vi "ConfigDlg.vi"(8 "error in (no error)":errorcluster, 11 "AnalysisPluginsBase in":refnum<class "AnalysisPluginsBase.lvclass">) -> (0 "error out":errorcluster, 2 "Changed":bool, 3 "AnalysisPluginsBase out":refnum<class "AnalysisPluginsBase.lvclass">)   [LabVIEW 2014, in "AnalysisPlugins.lvlib" / "AnalysisPluginsBase.lvclass"]
uses:
  AnalysisPluginsBase.lvclass
  Typedefs/clAnalysisConfig.ctl
  AnalysisPluginsBase.lvclass/AnalysisPluginsBase.ctl
  <userlib>/NIST/BaseClasses/BasePlugin_class/BasePlugin.lvclass/BasePlugin.ctl
  <userlib>/NIST/BaseClasses/BasePlugin_class/Accessors/Read PluginIniFilePath.vi
  Accessors/Write clConfig.vi
  Accessors/Read clConfig.vi
  Accessors/Read DelayCorr.vi
  Accessors/Read MagCorr.vi
  <vilib>/Utility/config.llb/NI_LVConfig.lvlib
panel:
  in  "BtnCancel":bool
  in  "MagCorr":dbl[](array[numeric])
  in  "DelayCorr":dbl[](array[numeric])
  in  "clAnalysisConfig":T1={"F0"=60, "SettlingTime"=7.0, "AnalysisCycles"=20.0, "SampleRate"=4800.0, "NumChannels"=6, "TsOffset"=enum."start"}
  in  "btnDone":bool
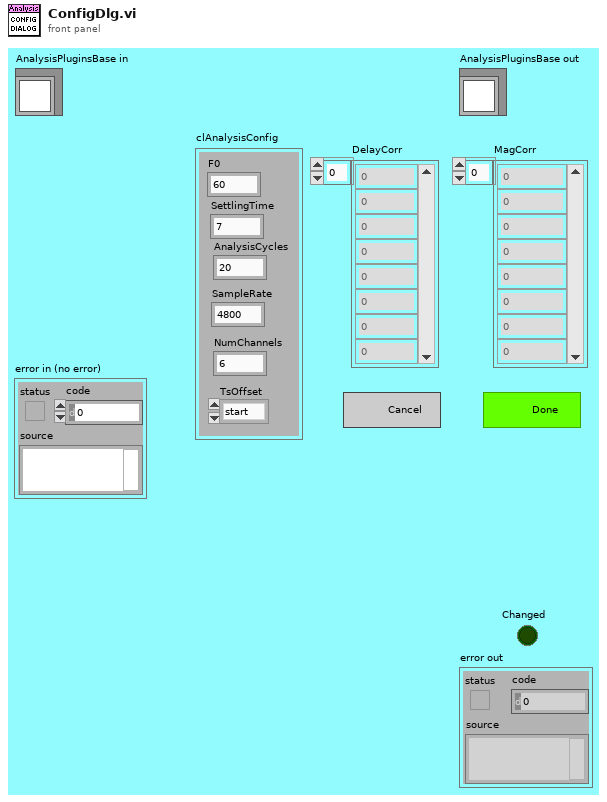
[diagram p1: front panel]
types:
  T1 = typedef "AnalysisPlugins.lvlib/AnalysisPluginsBase.lvclass/clAnalysisConfig.ctl" = cluster{"F0":u32, "SettlingTime":dbl, "AnalysisCycles":dbl, "SampleRate":dbl, "NumChannels":u32, "TsOffset":enum16{"start", "middle", "end"}}
  T2 = enum32{"Invalid", "Standard", "Closed", "Hidden", "Minimized", "Maximized"}
  T3 = enum32{"Invalid", "Default", "Floating", "Floating/Auto-Hide", "Modal"}
  T4 = typedef "NI_LVConfig.lvlib/Config Data RefNum.ctl" = refnum<k1>
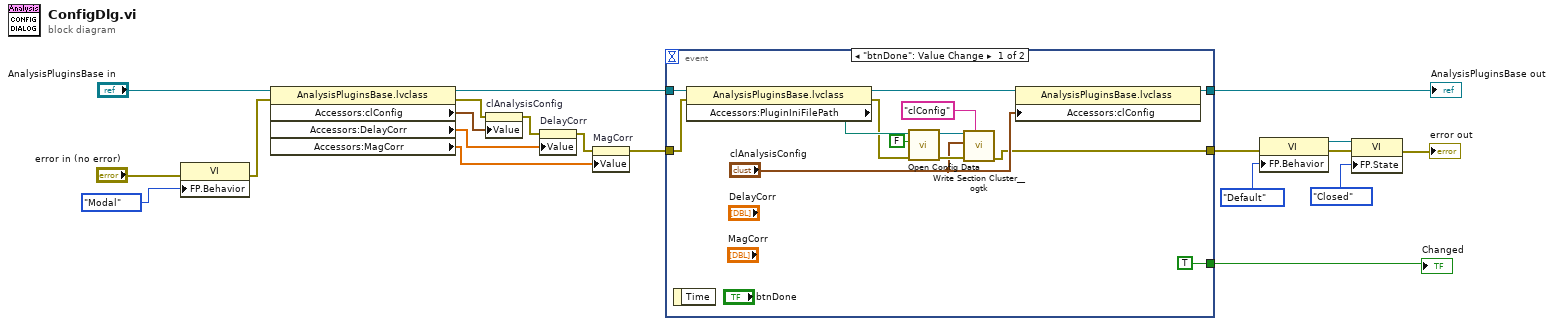
[diagram p0: block diagram]
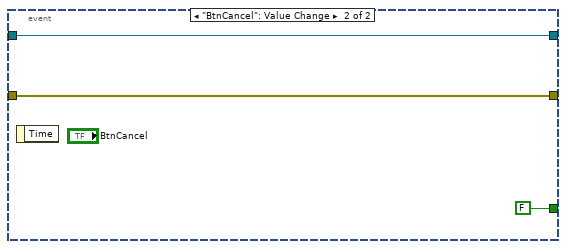
[diagram p2: hidden frame]
diagram:
  n1 = property class="VI"(error in="error in (no error)", "FP.Behavior"=T3."Modal" ("Front Panel Window:Behavior")) -> (error out=w7:errorcluster)  [unwired: 1 in, 1 out]
  n2 = property class="AnalysisPluginsBase.lvclass"(reference="AnalysisPluginsBase in", error in=w7) -> (reference out=w17:refnum<class "AnalysisPluginsBase.lvclass">, error out=w16:errorcluster, "Accessors:clConfig"=w15:T1, "Accessors:DelayCorr"=w14:dbl[], "Accessors:MagCorr"=w12:dbl[])
  n3 = property on="clAnalysisConfig" class="Clust (strict)"(error in=w16, "Value"=w15) -> (error out=w13:errorcluster)  [unwired: 1 in, 1 out]
  n4 = property on="DelayCorr" class="Arr (strict)"(error in=w13, "Value"=w14) -> (error out=w11:errorcluster)  [unwired: 1 in, 1 out]
  n5 = property on="MagCorr" class="Arr (strict)"(error in=w11, "Value"=w12) -> (error out=w10:errorcluster)  [unwired: 1 in, 1 out]
  n6 = event shown="[0] \"btnDone\": Value Change" {
    selector: _ -> [_ _]
    dyn-events: _ -> [_ _]
    timeout: _ -> [_ _]
    tunnel: [w23 w36] -> w19
    tunnel: w17 -> [w33 w36]
    tunnel: w10 -> [w28 w35]
    tunnel: [w21 w35] -> w6
    tunnel: [TRUE FALSE] -> w18
    event "btnDone": Value Change {
      n7 = event-data() -> ()  [unwired: 1 in, 1 out]
      n8 = property class="AnalysisPluginsBase.lvclass"(reference=w33, error in=w28) -> (reference out=w31:refnum<class "AnalysisPluginsBase.lvclass">, error out=w27:errorcluster, "Accessors:PluginIniFilePath"=w30:path)
      n9 = call <vilib>:"Open Config Data.vi"("error in (no error)"=w27, "create file if necessary (T)"=FALSE, "configuration file path"=w30) -> ("error out"=w25:errorcluster, "refnum"=w24:T4)  [unwired: 6 in, 1 out]
      n10 = call <userlib>:"Write Section Cluster__ogtk.vi"("section (optional)"="clConfig", "error in (no error)"=w25, "Section Formatted Cluster"="clAnalysisConfig", "refnum"=w24) -> ("error out"=w21:errorcluster)  [unwired: 6 in, 1 out]
      n11 = property class="AnalysisPluginsBase.lvclass"(reference=w31, "Accessors:clConfig"="clAnalysisConfig") -> (reference out=w23:refnum<class "AnalysisPluginsBase.lvclass">)  [unwired: 1 in, 1 out]
    }
    event "BtnCancel": Value Change {
      n12 = event-data() -> ()  [unwired: 1 in, 1 out]
    }
  }
  "AnalysisPluginsBase out" <- w19
  "Changed" <- w18
  n13 = property class="VI"(error in=w6, "FP.Behavior"=T3."Default" ("Front Panel Window:Behavior")) -> (reference out=w4:refnum<vi>, error out=w3:errorcluster)  [unwired: 1 in]
  n14 = property class="VI"(reference=w4, error in=w3, "FP.State"=T2."Closed" ("Front Panel Window:State")) -> (error out=→"error out":errorcluster)  [unwired: 1 out]
